vi "PH_Sound.Haenschen 1.vi"() -> (0 "Hänschen klein, ging allein, ...":cluster{"Tone":dbl, "Beats":i32}[](array[cluster]))   [LabVIEW 2009, in "PH_Sound.lvlib"]
doc: "\"Hänschen klein, ging alein, ...\""
uses:
  PH_Sound.lvlib
  PH_Common/PH_Audio/PH_3Oktaves.ctl
panel:
  out "size(s)":i32
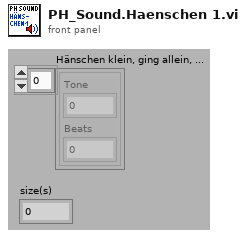
[diagram p1: front panel]
types:
  T1 = typedef "PH_3Oktaves.ctl" = dbl
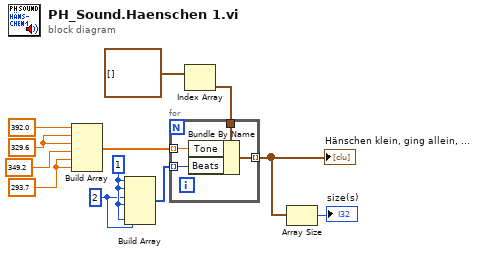
[diagram p0: block diagram]
diagram:
  w4 = u32 1 ("element")
  w3 = u32 2 ("y")
  w5 = T1 293.7 items=["c"=130.8, "cis"=138.6, "d"=146.8, "es"=155.6, "e"=164.8, "f"=174.6, "fis"=185.0, "g"=196.0, "as"=207.6, "a"=220.0, "b"=233.1, "h"=246.9, "c'"=261.6, "cis'"=277.2, "d'"=293.7, "es'"=311.1, "e'"=329.6, "f'"=349.2, "fis'"=370.0, "g'"=392.0, "as'"=415.3, "a'"=440.0, "b'"=466.2, "h'"=493.9, "c''"=523.3, "cis''"=554.4, "d''"=587.3, "es''"=622.3, "e''"=659.3, "f''"=689.5, "fis''"=740.0, "g''"=784.0, "as''"=830.6, "a''"=880.0, "b''"=932.3, "h''"=987.8, "c'''"=1047.0] ("3 Octaves")
  w6 = T1 349.2 items=["c"=130.8, "cis"=138.6, "d"=146.8, "es"=155.6, "e"=164.8, "f"=174.6, "fis"=185.0, "g"=196.0, "as"=207.6, "a"=220.0, "b"=233.1, "h"=246.9, "c'"=261.6, "cis'"=277.2, "d'"=293.7, "es'"=311.1, "e'"=329.6, "f'"=349.2, "fis'"=370.0, "g'"=392.0, "as'"=415.3, "a'"=440.0, "b'"=466.2, "h'"=493.9, "c''"=523.3, "cis''"=554.4, "d''"=587.3, "es''"=622.3, "e''"=659.3, "f''"=689.5, "fis''"=740.0, "g''"=784.0, "as''"=830.6, "a''"=880.0, "b''"=932.3, "h''"=987.8, "c'''"=1047.0] ("3 Octaves")
  w7 = T1 329.6 items=["c"=130.8, "cis"=138.6, "d"=146.8, "es"=155.6, "e"=164.8, "f"=174.6, "fis"=185.0, "g"=196.0, "as"=207.6, "a"=220.0, "b"=233.1, "h"=246.9, "c'"=261.6, "cis'"=277.2, "d'"=293.7, "es'"=311.1, "e'"=329.6, "f'"=349.2, "fis'"=370.0, "g'"=392.0, "as'"=415.3, "a'"=440.0, "b'"=466.2, "h'"=493.9, "c''"=523.3, "cis''"=554.4, "d''"=587.3, "es''"=622.3, "e''"=659.3, "f''"=689.5, "fis''"=740.0, "g''"=784.0, "as''"=830.6, "a''"=880.0, "b''"=932.3, "h''"=987.8, "c'''"=1047.0] ("3 Octaves")
  w8 = T1 392.0 items=["c"=130.8, "cis"=138.6, "d"=146.8, "es"=155.6, "e"=164.8, "f"=174.6, "fis"=185.0, "g"=196.0, "as"=207.6, "a"=220.0, "b"=233.1, "h"=246.9, "c'"=261.6, "cis'"=277.2, "d'"=293.7, "es'"=311.1, "e'"=329.6, "f'"=349.2, "fis'"=370.0, "g'"=392.0, "as'"=415.3, "a'"=440.0, "b'"=466.2, "h'"=493.9, "c''"=523.3, "cis''"=554.4, "d''"=587.3, "es''"=622.3, "e''"=659.3, "f''"=689.5, "fis''"=740.0, "g''"=784.0, "as''"=830.6, "a''"=880.0, "b''"=932.3, "h''"=987.8, "c'''"=1047.0] ("3 Octaves")
  n1 = Build Array(w8, w7, w7, w6, w5, w5) -> (w2:T1[])
  n2 = Build Array(w4, w4, w3, w4, w4, w3) -> (w1:u32[])
  n3 = Index Array(array=cluster{"Tone":dbl, "Beats":i32}[] [] ("Song")) -> (element=w9:cluster{"Tone":dbl, "Beats":i32})  [unwired: 1 in]
  n4 = for {
    tunnel: w2 -> [w15] mode=indexing
    tunnel: w1 -> [w14] mode=indexing
    tunnel: w9 -> [w16]
    tunnel: [w13] -> w12 mode=indexing
    n5 = Bundle By Name(cluster=w16, "Tone"=w15, "Beats"=w14) -> (w13:cluster{"Tone":dbl, "Beats":i32})
  }
  "Hänschen klein, ging allein, ..." <- w12
  n6 = Array Size(array=w12) -> (size(s)=→"size(s)":i32)
